vi "waveformprepareRFcoil.vi"(6 "RF pulse length (Units 1us)":dbl=1000.0, 9 "1762 pulse length (units of 1 us)":dbl=50.0) -> (3 "digital waveform out 2":digitalwaveform(waveform)={"t0"=timestamp(0 s since 1904-01-01), "dt"=1e-07, "Y"={"transitions"=[0, 2100, 2200, 2300, 2351, 2401, 2451, 2551], "data"=[[0, 1, 1, 1, 0, 0], [0, 1, 0, 1, 0, 0], [0, 1, 0, 0, 0, 0], [0, 0, 0, 0, 0, 0], [1, 0, 0, 0, 0, 0], [0, 0, 0, 0, 0, 1], [0, 0, 0, 0, 0, 0], [0, 0, 1, 1, 0, 0]]}, "error"={"status"=FALSE, "code"=37421928, "source"=""}})   [LabVIEW 2012]
uses:
  <vilib>/Waveform/DWDTOps.llb/Digital Pattern Generator (Single Value).vi
  <vilib>/Waveform/DWDTOps.llb/DWDT Append Digital Samples.vi
panel:
  out "Mixed Signal Graph":digitalwaveform(graph)={"t0"=timestamp(0 s since 1904-01-01), "dt"=1e-07, "Y"={"transitions"=[0, 2100, 2200, 2300, 2351, 2401, 2451, 2551], "data"=[[0, 1, 1, 1, 0, 0], [0, 1, 0, 1, 0, 0], [0, 1, 0, 0, 0, 0], [0, 0, 0, 0, 0, 0], [1, 0, 0, 0, 0, 0], [0, 0, 0, 0, 0, 1], [0, 0, 0, 0, 0, 0], [0, 0, 1, 1, 0, 0]]}, "error"={"status"=FALSE, "code"=37421928, "source"=""}}
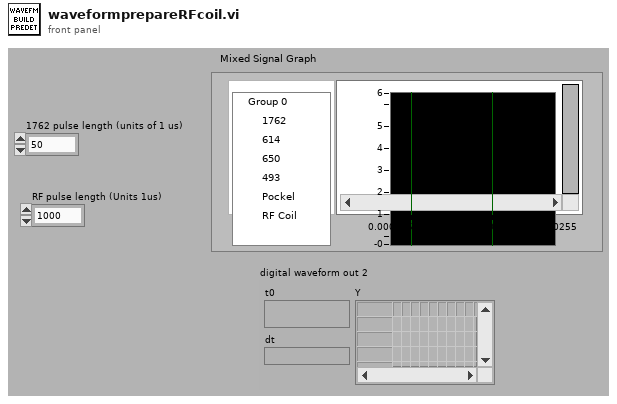
[diagram p1: front panel]
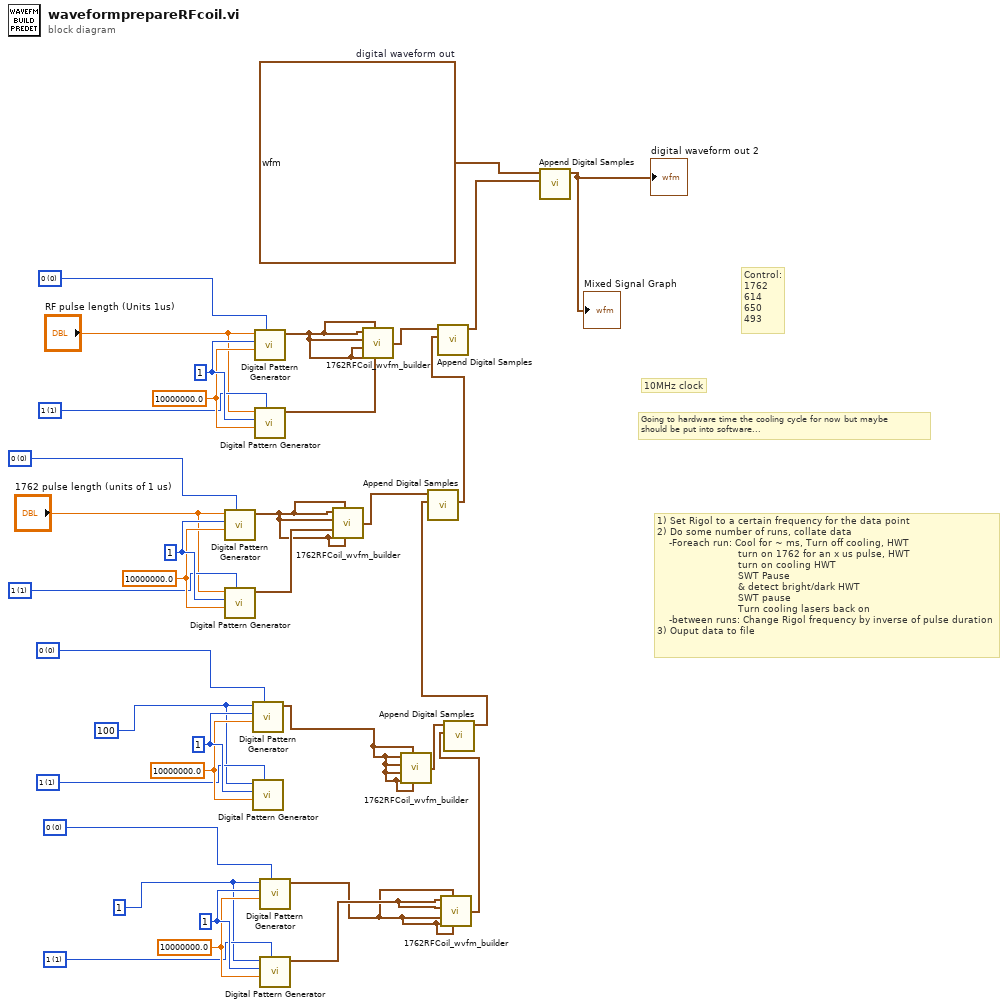
[diagram p0: block diagram]
diagram:
  w10 = u8 0 items=["0", "1", "Z", "L", "H", "X", "T", "V"] ("value")
  w9 = u32 1 ("number of signals")
  w7 = u8 1 items=["0", "1", "Z", "L", "H", "X", "T", "V"] ("value")
  w8 = 10000000.0 ("rate")
  w20 = u32 1 ("number of samples")
  w24 = u8 0 items=["0", "1", "Z", "L", "H", "X", "T", "V"] ("value")
  w23 = u32 1 ("number of signals")
  w21 = u8 1 items=["0", "1", "Z", "L", "H", "X", "T", "V"] ("value")
  w22 = 10000000.0 ("rate")
  w25 = u32 100 ("number of samples")
  w29 = u8 0 items=["0", "1", "Z", "L", "H", "X", "T", "V"] ("value")
  w28 = u32 1 ("number of signals")
  w26 = u8 1 items=["0", "1", "Z", "L", "H", "X", "T", "V"] ("value")
  w27 = 10000000.0 ("rate")
  w36 = u8 0 items=["0", "1", "Z", "L", "H", "X", "T", "V"] ("value")
  w35 = u32 1 ("number of signals")
  w33 = u8 1 items=["0", "1", "Z", "L", "H", "X", "T", "V"] ("value")
  w34 = 10000000.0 ("rate")
  w30 = digitalwaveform {"t0"=timestamp(0 s since 1904-01-01), "dt"=1e-07, "Y"={"transitions"=[0, 2100, 2200, 2300, 2350], "data"=[[0, 1, 1, 1, 0, 0], [0, 1, 0, 1, 0, 0], [0, 1, 0, 0, 0, 0], [0, 0, 0, 0, 0, 0], [0, 0, 0, 0, 0, 0]]}, "error"={"status"=FALSE, "code"=37421928, "source"=""}}  # digital waveform out
  # "Going to hardware time the cooling cycle for now but maybe\nshould be put into software..."
  # "10MHz clock"
  # "Control:\n1762\n614\n650\n493"
  # "1) Set Rigol to a certain frequency for the data point\n2) Do some number of runs, collate data\n    -Foreach run: Cool for ~ ms, Turn off cooling, HWT\n                           turn on 1762 for an x us pulse, HWT\n                           turn on cooling HWT\n                           SWT Pause\n                           & detect bright/dark HWT\n                           SWT pause\n                           Turn cooling lasers back on \n    -between runs: Change Rigol frequency by inverse of pulse duration\n3) Ouput data to file"
  n1 = call-poly <vilib>:"Digital Pattern Generator.vi"("value"=w36, "sample rate"=w34, "number of signals"=w35, "number of samples"="1762 pulse length (units of 1 us)") -> ("digital waveform"=w13:digitalwaveform)  [unwired: 6 in, 1 out]
  n2 = call-poly <vilib>:"Digital Pattern Generator.vi"("value"=w33, "sample rate"=w34, "number of signals"=w35, "number of samples"="1762 pulse length (units of 1 us)") -> ("digital waveform"=w14:digitalwaveform)  [unwired: 6 in, 1 out]
  n3 = call-poly <vilib>:"Digital Pattern Generator.vi"("value"=w29, "sample rate"=w27, "number of signals"=w28, "number of samples"=w25) -> ("digital waveform"=w12:digitalwaveform)  [unwired: 6 in, 1 out]
  n4 = call-poly <vilib>:"Digital Pattern Generator.vi"("value"=w26, "sample rate"=w27, "number of signals"=w28, "number of samples"=w25) -> ()  [unwired: 6 in, 2 out]
  n5 = call-poly <vilib>:"Digital Pattern Generator.vi"("value"=w10, "sample rate"=w8, "number of signals"=w9, "number of samples"="RF pulse length (Units 1us)") -> ("digital waveform"=w2:digitalwaveform)  [unwired: 6 in, 1 out]
  n6 = call-poly <vilib>:"Digital Pattern Generator.vi"("value"=w7, "sample rate"=w8, "number of signals"=w9, "number of samples"="RF pulse length (Units 1us)") -> ("digital waveform"=w1:digitalwaveform)  [unwired: 6 in, 1 out]
  n7 = call-poly <vilib>:"Digital Pattern Generator.vi"("value"=w24, "sample rate"=w22, "number of signals"=w23, "number of samples"=w20) -> ("digital waveform"=w11:digitalwaveform)  [unwired: 6 in, 1 out]
  n8 = call-poly <vilib>:"Digital Pattern Generator.vi"("value"=w21, "sample rate"=w22, "number of signals"=w23, "number of samples"=w20) -> ("digital waveform"=w16:digitalwaveform)  [unwired: 6 in, 1 out]
  n9 = call "1762RFCoil_wvfm_builder.vi"("RFCoil"=w13, "pockel"=w13, "614"=w13, "1762"=w14, "650"=w13, "493"=w13) -> ("out"=w18:digitalwaveform)
  n10 = call "1762RFCoil_wvfm_builder.vi"("RFCoil"=w1, "pockel"=w2, "614"=w2, "1762"=w2, "650"=w2, "493"=w2) -> ("out"=w5:digitalwaveform)
  n11 = call "1762RFCoil_wvfm_builder.vi"("RFCoil"=w12, "pockel"=w12, "614"=w12, "1762"=w12, "650"=w12, "493"=w12) -> ("out"=w17:digitalwaveform)
  n12 = call "1762RFCoil_wvfm_builder.vi"("RFCoil"=w11, "pockel"=w11, "614"=w11, "1762"=w11, "650"=w16, "493"=w16) -> ("out"=w15:digitalwaveform)
  n13 = call-poly <vilib>:"Append Digital Samples.vi"("digital waveform B"=w15, "digital waveform A"=w17) -> ("digital waveform out"=w19:digitalwaveform)  [unwired: 8 in, 1 out]
  n14 = call-poly <vilib>:"Append Digital Samples.vi"("digital waveform B"=w19, "digital waveform A"=w18) -> ("digital waveform out"=w4:digitalwaveform)  [unwired: 8 in, 1 out]
  n15 = call-poly <vilib>:"Append Digital Samples.vi"("digital waveform B"=w4, "digital waveform A"=w5) -> ("digital waveform out"=w3:digitalwaveform)  [unwired: 8 in, 1 out]
  n16 = call-poly <vilib>:"Append Digital Samples.vi"("digital waveform B"=w3, "digital waveform A"=w30) -> ("digital waveform out"=→"Mixed Signal Graph" →"digital waveform out 2":digitalwaveform)  [unwired: 8 in, 1 out]
